vi "Save Recipe.vi"(8 "error in (no error)":errorcluster, 10 "Control Panel":T1 {"Unit" items=["mm", "inch"]}, 11 "Master in":refnum<class "Master.lvclass">) -> (0 "error out":errorcluster, 3 "Master out":refnum<class "Master.lvclass">, 4 "Save":bool)   [LabVIEW 2014, in "Master.lvclass"]
uses:
  Master/Master.lvclass
  Master/Master.lvclass/Master.ctl
panel:
  # "RPS"
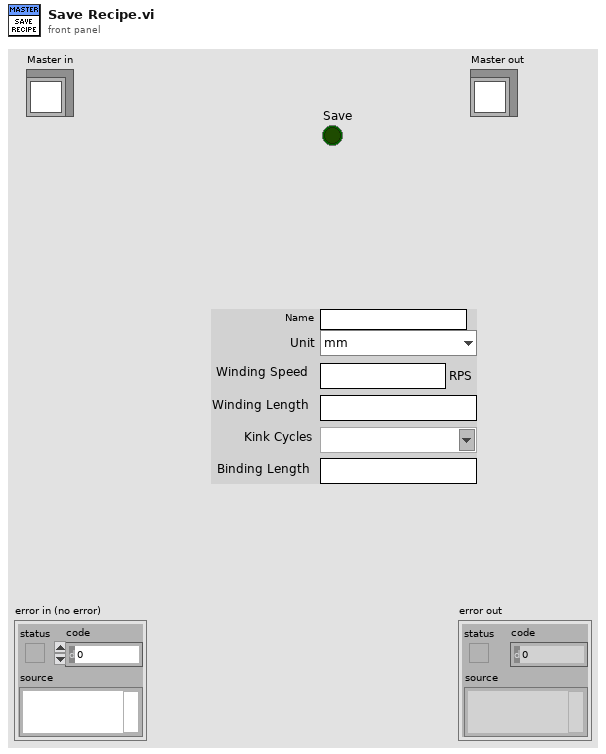
[diagram p1: front panel]
types:
  T1 = cluster{"Name":string, "Unit":u16, "Winding Speed":string, "Winding Length":string, "Kink Cycles":string, "Binding Length":string}
  T2 = cluster{"Name":string, "Winding Length":string, "Winding Speed":string, "Kink Cycles":string, "Binding Length":string, "Unit":string}
  T3 = cluster{"Para":cluster{"Name":string, "Wind Length":string, "Wind Spd":string, "Kink Cyc":string, "Bind Length":string, "Unit":string}[]}
  T4 = cluster{"Name":string, "Wind Length":string, "Wind Spd":string, "Kink Cyc":string, "Bind Length":string, "Unit":string}[]
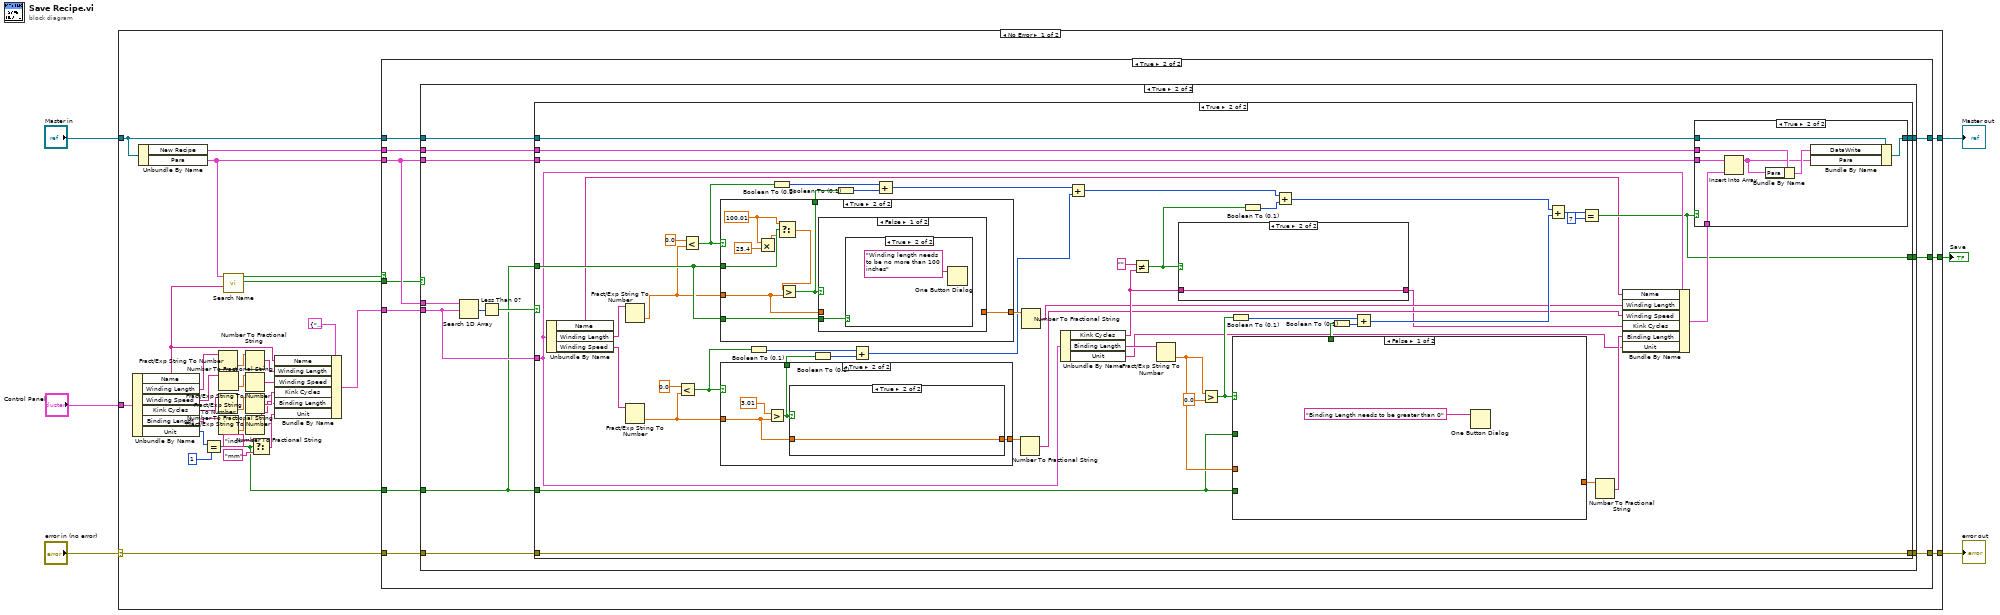
[diagram p0: block diagram]
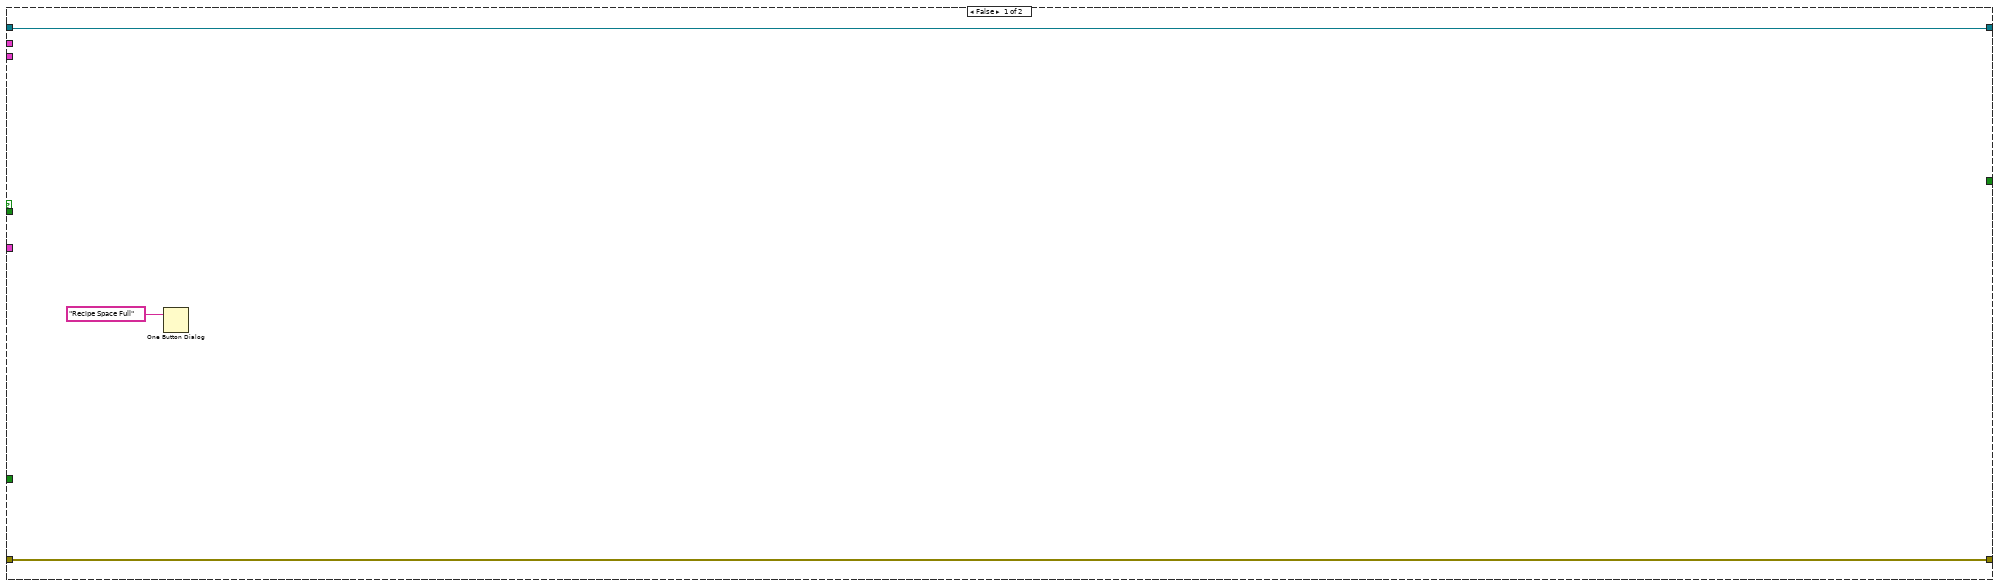
[diagram p2: hidden frame]
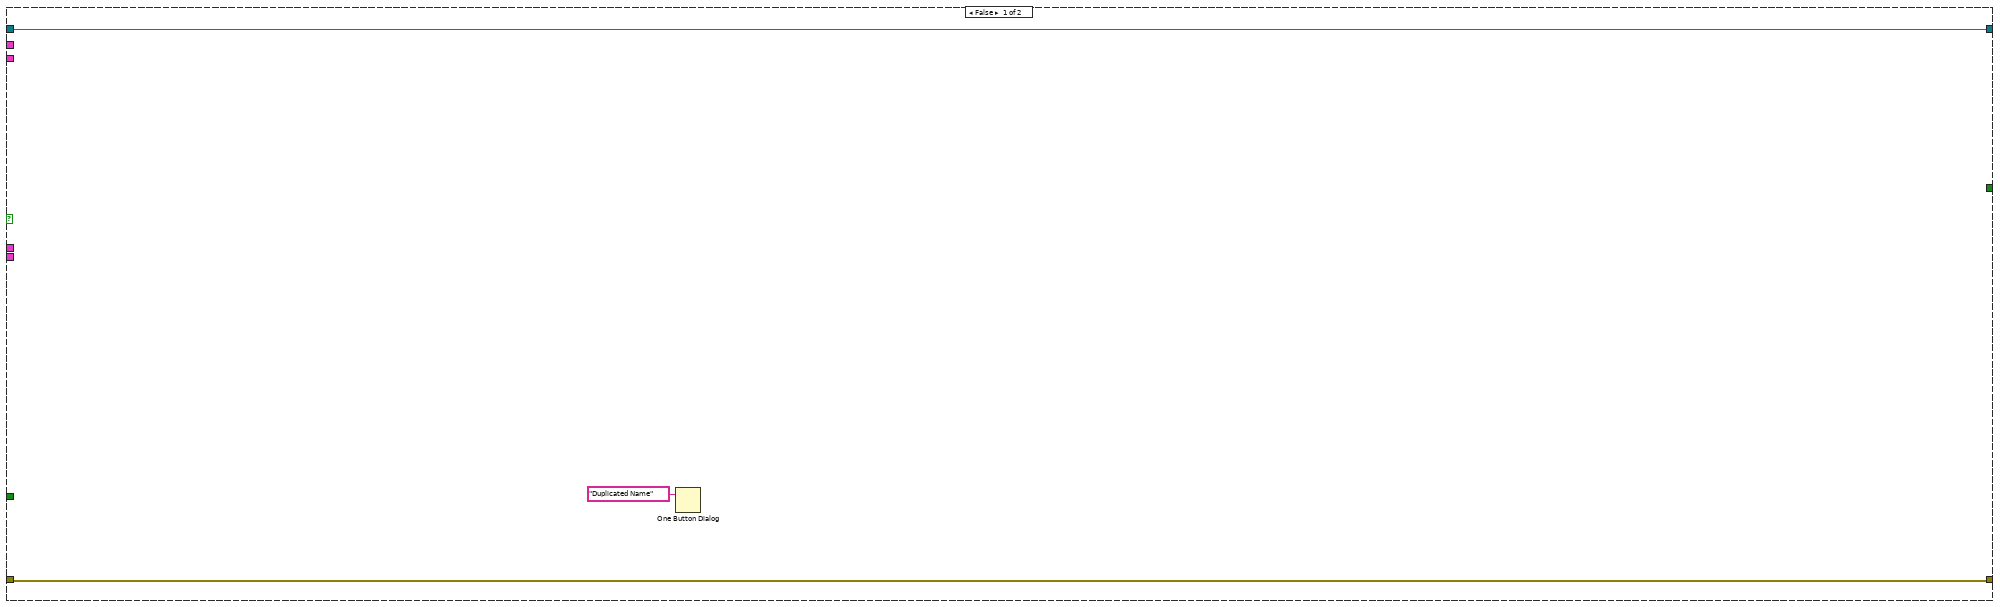
[diagram p3: hidden frame]
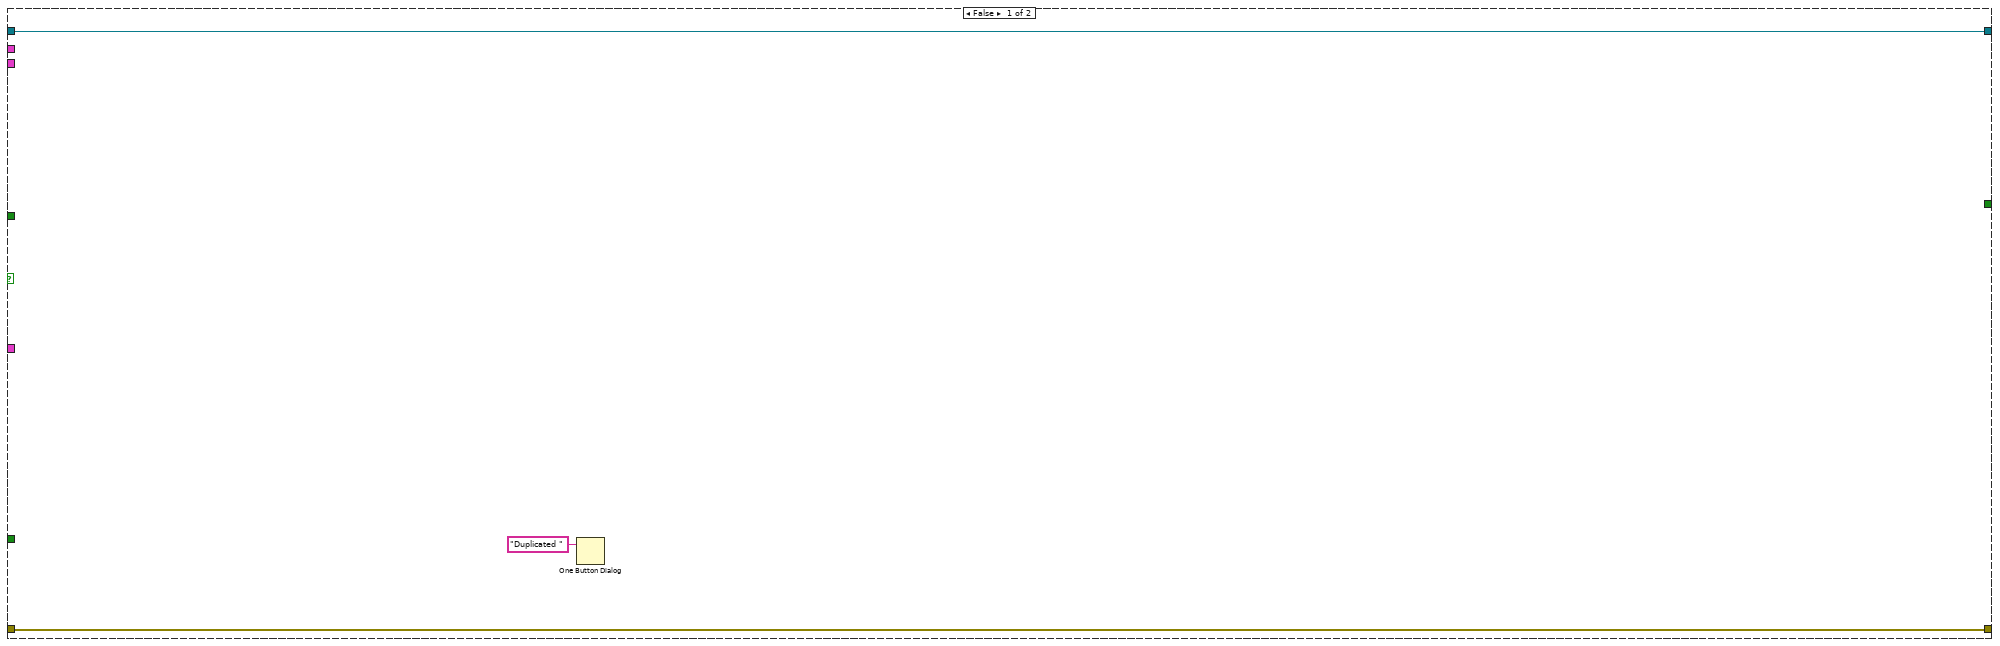
[diagram p4: hidden frame]
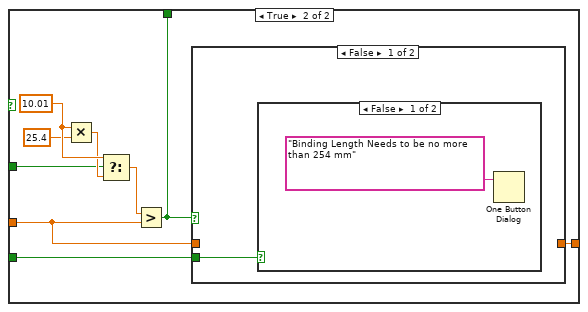
[diagram p5: hidden frame]
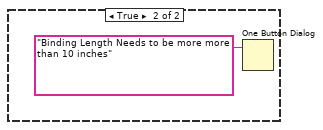
[diagram p6: hidden frame]
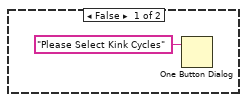
[diagram p8: hidden frame]
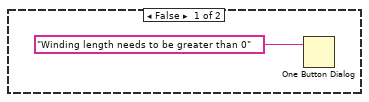
[diagram p9: hidden frame]
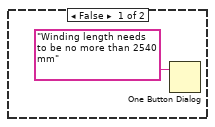
[diagram p10: hidden frame]
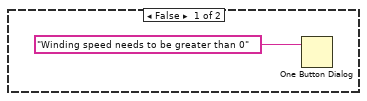
[diagram p12: hidden frame]
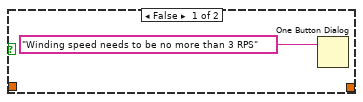
[diagram p13: hidden frame]
diagram:
  n1 = case shown="No Error" "error in (no error)" {
    selector: "error in (no error)" -> [w37 w166]
    tunnel: [w15 w166] -> w5
    tunnel: [w16 w165] -> w3
    tunnel: "Master in" -> [w11 w165]
    tunnel: "Control Panel" -> [w24 _]
    tunnel: [w12 _] -> w1
    frame No Error {
      n2 = Unbundle By Name(w24) -> ("Name"=w7:string, "Winding Length"=w28:string, "Winding Speed"=w27:string, "Kink Cycles"=w26:string, "Binding Length"=w25:string, "Unit"=w33:u16)
      n3 = Unbundle By Name(w11) -> ("New Recipe"=w14:T3, "Para"=w9:T4)
      n4 = Equal?(x=w33, y=u16 1) -> (x = y?=w13:bool)
      n5 = Fract/Exp String To Number(string=w28) -> (number=w29:dbl)  [unwired: 3 in, 1 out]
      n6 = Fract/Exp String To Number(string=w26) -> (number=w35:dbl)  [unwired: 3 in, 1 out]
      n7 = Fract/Exp String To Number(string=w27) -> (number=w30:dbl)  [unwired: 3 in, 1 out]
      n8 = Fract/Exp String To Number(string=w25) -> (number=w36:dbl)  [unwired: 3 in, 1 out]
      n9 = call "Search Name.vi"("element"=w7, "New Recipe.Para"=w9) -> ("x < 0?"=w10:bool, "x = y?"=w8:bool)  [unwired: 8 in]
      n10 = Number To Fractional String(number=w29) -> (F-format string=w22:string)  [unwired: 3 in]
      n11 = Number To Fractional String(number=w30) -> (F-format string=w21:string)  [unwired: 3 in]
      n12 = Number To Fractional String(number=w35) -> (F-format string=w20:string)  [unwired: 3 in]
      n13 = Number To Fractional String(number=w36) -> (F-format string=w19:string)  [unwired: 3 in]
      n14 = Select(t="inch", s=w13, f="mm") -> (s? t:f=w17:string)
      n15 = Bundle By Name(cluster=T2 {"Name"="", "Winding Length"="", "Winding Speed"="", "Kink Cycles"="", "Binding Length"="", "Unit"=""}, "Name"=w7, "Winding Length"=w22, "Winding Speed"=w21, "Kink Cycles"=w20, "Binding Length"=w19, "Unit"=w17) -> (w23:T2)
      n16 = case shown="True" w8 {
        tunnel: w37 -> [w40 w48]
        tunnel: [w40 w49] -> w15
        tunnel: w9 -> [_ w45]
        tunnel: w23 -> [_ w50]
        tunnel: [w38 w46] -> w16
        tunnel: w11 -> [w38 w47]
        tunnel: w14 -> [_ w44]
        tunnel: w13 -> [_ w43]
        tunnel: [_ w42] -> w12
        tunnel: w10 -> [_ w41]
        frame False {
          n17 = One Button Dialog(message="Recipe Space Full") -> ()  [unwired: 1 in, 1 out]
        }
        frame True {
          n18 = case shown="True" w41 {
            tunnel: w45 -> [_ w64]
            tunnel: w50 -> [_ w56]
            tunnel: [w52 w60] -> w49
            tunnel: w48 -> [w52 w61]
            tunnel: [w51 w62] -> w46
            tunnel: w47 -> [w51 w63]
            tunnel: w45 -> [_ w58]
            tunnel: w44 -> [_ w57]
            tunnel: w43 -> [_ w55]
            tunnel: [_ w54] -> w42
            frame False {
              n19 = One Button Dialog(message="Duplicated Name") -> ()  [unwired: 1 in, 1 out]
            }
            frame True {
              n20 = Search 1D Array(1D array=w64, element=w56) -> (index of element=w65:i32)  [unwired: 1 in]
              n21 = Less Than 0?(x=w65) -> (x < 0?=w59:bool)
              n22 = case shown="True" w59 {
                tunnel: w63 -> [w66 w117]
                tunnel: [w66 w118] -> w62
                tunnel: w61 -> [w67 w119]
                tunnel: [w67 w119] -> w60
                tunnel: w58 -> [_ w116]
                tunnel: w57 -> [_ w115]
                tunnel: w56 -> [_ w77]
                tunnel: w55 -> [_ w106]
                tunnel: w55 -> [_ w92]
                tunnel: [_ w70] -> w54
                frame False {
                  n23 = One Button Dialog(message="Duplicated ") -> ()  [unwired: 1 in, 1 out]
                }
                frame True {
                  n24 = Unbundle By Name(w77) -> ("Name"=w69:string, "Winding Length"=w107:string, "Winding Speed"=w108:string)
                  n25 = Fract/Exp String To Number(string=w107) -> (number=w102:dbl)  [unwired: 3 in, 1 out]
                  n26 = Fract/Exp String To Number(string=w108) -> (number=w113:dbl)  [unwired: 3 in, 1 out]
                  n27 = Less?(x=0.0, y=w113) -> (x < y?=w109:bool)
                  n28 = Less?(x=0.0, y=w102) -> (x < y?=w101:bool)
                  n29 = case shown="True" w101 {
                    tunnel: [_ w145] -> w100
                    tunnel: w102 -> [_ w144]
                    tunnel: [_ w143] -> w99
                    tunnel: w106 -> [_ w142]
                    tunnel: w106 -> [_ w137]
                    frame False {
                      n30 = One Button Dialog(message="Winding length needs to be greater than 0") -> ()  [unwired: 1 in, 1 out]
                    }
                    frame True {
                      w139 = 100.01 ("x")
                      n31 = Multiply(x=w139, y=25.4) -> (x*y=w138:dbl)
                      n32 = Select(t=w139, s=w142, f=w138) -> (s? t:f=w141:dbl)
                      n33 = Greater?(x=w141, y=w144) -> (0:w145:bool)
                      n34 = case shown="False" w145 {
                        tunnel: w144 -> [_ w149]
                        tunnel: [_ w149] -> w143
                        tunnel: w137 -> [w146 _]
                        frame False {
                          n35 = case shown="True" w146 {
                            frame False {
                              n36 = One Button Dialog(message="Winding length needs to be no more than 2540 mm") -> ()  [unwired: 1 in, 1 out]
                            }
                            frame True {
                              n37 = One Button Dialog(message="Winding length needs to be no more than 100 inches") -> ()  [unwired: 1 in, 1 out]
                            }
                          }
                        }
                        frame True {
                        }
                      }
                    }
                  }
                  n38 = case shown="True" w109 {
                    tunnel: w113 -> [_ w153]
                    tunnel: [_ w152] -> w98
                    tunnel: [_ w151] -> w110
                    frame False {
                      n39 = One Button Dialog(message="Winding speed needs to be greater than 0") -> ()  [unwired: 1 in, 1 out]
                    }
                    frame True {
                      n40 = Greater?(x=3.01, y=w153) -> (0:w151:bool)
                      n41 = case shown="True" w151 {
                        tunnel: w153 -> [_ w156]
                        tunnel: [_ w156] -> w152
                        frame False {
                          n42 = One Button Dialog(message="Winding speed needs to be no more than 3 RPS") -> ()  [unwired: 1 in, 1 out]
                        }
                        frame True {
                        }
                      }
                    }
                  }
                  n43 = Boolean To (0,1)(Boolean=w109) -> (0, 1=w111:i16)
                  n44 = Boolean To (0,1)(Boolean=w101) -> (0, 1=w104:i16)
                  n45 = Boolean To (0,1)(Boolean=w110) -> (0, 1=w112:i16)
                  n46 = Boolean To (0,1)(Boolean=w100) -> (0, 1=w105:i16)
                  n47 = Add(x=w111, y=w112) -> (x+y=w84:i16)
                  n48 = Add(x=w104, y=w105) -> (x+y=w85:i16)
                  n49 = Number To Fractional String(number=w98) -> (F-format string=w75:string)  [unwired: 3 in]
                  n50 = Number To Fractional String(number=w99) -> (F-format string=w76:string)  [unwired: 3 in]
                  n51 = Unbundle By Name(w77) -> ("Kink Cycles"=w95:string, "Binding Length"=w97:string, "Unit"=w72:string)
                  n52 = Add(x=w85, y=w84) -> (x+y=w83:i16)
                  n53 = Not Equal?(x="", y=w95) -> (x != y?=w91:bool)
                  n54 = Fract/Exp String To Number(string=w97) -> (number=w93:dbl)  [unwired: 3 in, 1 out]
                  n55 = case shown="True" w91 {
                    tunnel: [_ w135] -> w74
                    tunnel: w95 -> [_ w135]
                    frame False {
                      n56 = One Button Dialog(message="Please Select Kink Cycles") -> ()  [unwired: 1 in, 1 out]
                    }
                    frame True {
                    }
                  }
                  n57 = Greater?(x=w93, y=0.0 ("x")) -> (0:w87:bool)
                  n58 = Boolean To (0,1)(Boolean=w87) -> (0, 1=w89:i16)
                  n59 = case shown="False" w87 {
                    tunnel: w93 -> [_ w129]
                    tunnel: [_ w127] -> w86
                    tunnel: [_ w128] -> w88
                    tunnel: w92 -> [_ w123]
                    tunnel: w92 -> [_ w121]
                    frame False {
                      n60 = One Button Dialog(message="Binding Length needs to be greater than 0") -> ()  [unwired: 1 in, 1 out]
                    }
                    frame True {
                      w126 = 10.01 ("x")
                      n61 = Multiply(x=w126, y=25.4) -> (x*y=w124:dbl)
                      n62 = Select(t=w126, s=w123, f=w124) -> (s? t:f=w122:dbl)
                      n63 = Greater?(x=w122, y=w129) -> (0:w128:bool)
                      n64 = case shown="False" w128 {
                        tunnel: w129 -> [_ w133]
                        tunnel: [_ w133] -> w127
                        tunnel: w121 -> [w130 _]
                        frame False {
                          n65 = case shown="False" w130 {
                            frame False {
                              n66 = One Button Dialog(message="Binding Length Needs to be no more than 254 mm") -> ()  [unwired: 1 in, 1 out]
                            }
                            frame True {
                              n67 = One Button Dialog(message="Binding Length Needs to be more more than 10 inches") -> ()  [unwired: 1 in, 1 out]
                            }
                          }
                        }
                        frame True {
                        }
                      }
                    }
                  }
                  n68 = Boolean To (0,1)(Boolean=w91) -> (0, 1=w82:i16)
                  n69 = Add(x=w83, y=w82) -> (x+y=w81:i16)
                  n70 = Boolean To (0,1)(Boolean=w88) -> (0, 1=w90:i16)
                  n71 = Add(x=w89, y=w90) -> (x+y=w80:i16)
                  n72 = Add(x=w81, y=w80) -> (x+y=w79:i16)
                  n73 = Equal?(x=w79, y=i16 7) -> (x = y?=w70:bool)
                  n74 = Number To Fractional String(number=w86) -> (F-format string=w73:string)  [unwired: 3 in]
                  n75 = Bundle By Name(cluster=w77, "Name"=w69, "Winding Length"=w76, "Winding Speed"=w75, "Kink Cycles"=w74, "Binding Length"=w73, "Unit"=w72) -> (w71:T2)
                  n76 = case shown="True" w70 {
                    tunnel: w116 -> [_ w164]
                    tunnel: w117 -> [w157 w163]
                    tunnel: [w157 w162] -> w118
                    tunnel: w115 -> [_ w161]
                    tunnel: w71 -> [_ w158]
                    frame False {
                    }
                    frame True {
                      n77 = Insert Into Array(array=w164, new element=w158) -> (w159:T4)  [unwired: 1 in]
                      n78 = Bundle By Name(cluster=w161, "Para"=w159) -> (w160:T3)
                      n79 = Bundle By Name(cluster=w163, "DataWrite"=w160, "Para"=w159) -> (w162:refnum<class "Master.lvclass">)
                    }
                  }
                }
              }
            }
          }
        }
      }
    }
    frame Error {
    }
  }
  "error out" <- w5
  "Master out" <- w3
  "Save" <- w1
